vi "Open.vi"(8 "error in (no error)":errorcluster, 11 "MelsecTCP in":refnum<class "Abstract PLC Controler.lvclass">) -> (0 "error out":errorcluster, 3 "MelsecTCP out":refnum<class "Abstract PLC Controler.lvclass">)   [LabVIEW 2020, in "HslCommunication.lvlib" / "Abstract PLC Controler.lvclass"]
uses:
  Abstract PLC Controler.lvclass
  EventLogger.lvlibp/1abvi3w/vi.lib/gpm_packages/@cs/event-logger/Source/Composed Log/Types/Log Level.ctl
  Abstract PLC Controler.lvclass/Abstract PLC Controler.ctl
  EventLogger.lvlibp/Logger.lvclass
  EventLogger.lvlibp/1abvi3w/vi.lib/gpm_packages/@cs/event-logger/Source/Composed Log/Composed Log.lvlib
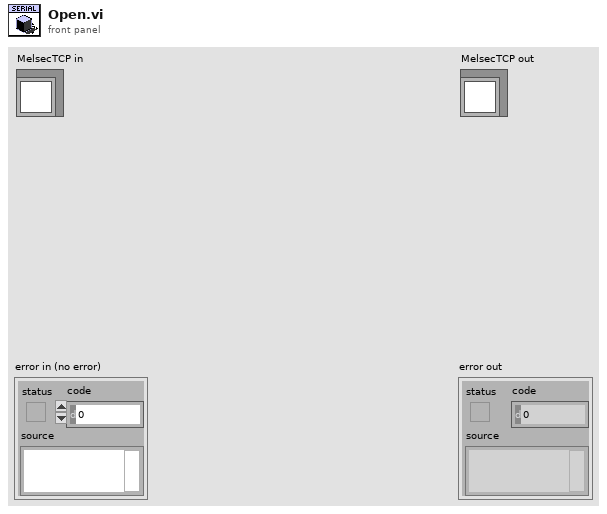
[diagram p1: front panel]
types:
  T1 = typedef "EventLogger.lvlibp/Composed Log.lvlib/Log Level.ctl" = enum16{"Debug", "Info", "Warning", "Error", "Critical"}
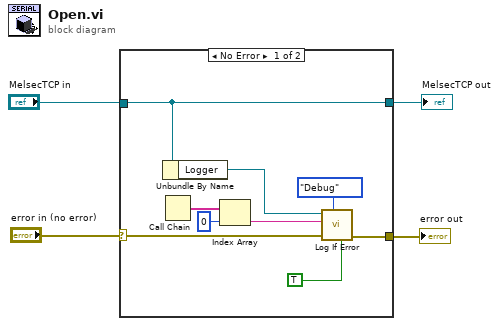
[diagram p0: block diagram]
diagram:
  n1 = case shown="No Error" "error in (no error)" {
    selector: "error in (no error)" -> [w13 w15]
    tunnel: [w12 w15] -> w3
    tunnel: "MelsecTCP in" -> [w5 w14]
    tunnel: [w5 w14] -> w1
    frame No Error {
      n2 = Unbundle By Name(w5) -> ("Logger"=w11:refnum<class "Logger.lvclass">)
      n3 = Call Chain() -> (call chain=w9:string[])
      n4 = Index Array(array=w9, index=0) -> (element=w7:string)
      n5 = call "Log If Error.vi"("Include Warnings(F)"=TRUE, "Event Level (Error)"=Log_Level."Debug", "error in (no error)"=w13, "SourceID"=w7, "Logger in"=w11) -> ("error out"=w12:errorcluster)  [unwired: 5 in, 1 out]
    }
    frame Error {
    }
  }
  "error out" <- w3
  "MelsecTCP out" <- w1
